vi "Query Max Current Limit.vi"(8 "error in (no error)":errorcluster, 9 "voltage level (0.0 Volts)":dbl[unit] format="%^.2e", 10 "channel name (\"CHANNEL1\")":string="CHANNEL1", 11 "IVI_DCPwr in":refnum<class "IVI_DCPwr.lvclass">) -> (0 "error out":errorcluster, 2 "max current limit":dbl[unit] format="%^.2e", 3 "IVI_DCPwr out":refnum<class "IVI_DCPwr.lvclass">)   [LabVIEW 2013, in "IVI_DCPwr.lvlib" / "IVI_DCPwr.lvclass"]
doc: "This VI returns the maximum programmable current limit that the power supply accepts for a particular voltage level on a channel for the output range to which the power supply is currently configured."
uses:
  IVI_DCPwr.lvclass
  IVI_DCPwr.lvclass/IVI_DCPwr.ctl
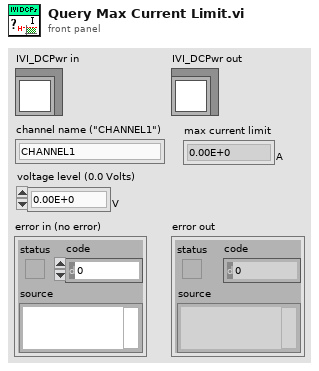
[diagram p1: front panel]
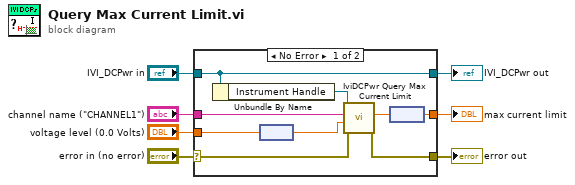
[diagram p0: block diagram]
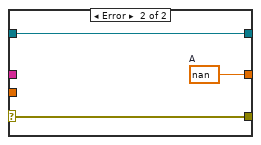
[diagram p2: hidden frame]
diagram:
  n1 = case shown="No Error" "error in (no error)" {
    selector: "error in (no error)" -> [w14 w19]
    tunnel: [w13 w19] -> w6
    tunnel: [w16 w18] -> w4
    tunnel: "IVI_DCPwr in" -> [w16 w18]
    tunnel: "channel name (\"CHANNEL1\")" -> [w12 _]
    tunnel: [w8 w17] -> w1
    tunnel: "voltage level (0.0 Volts)" -> [w10 _]
    frame No Error {
      n2 = Unbundle By Name(w16) -> ("Instrument Handle"=w15:refnum<k15>)
      n3 = node(w10) -> (w9:dbl)
      n4 = call <vilib>:"IviDCPwr Query Max Current Limit.vi"("error in (no error)"=w14, "voltage level (0.0 Volts)"=w9, "channel name (\"CHANNEL1\")"=w12, "instrument handle"=w15) -> ("error out"=w13:errorcluster, "max current limit"=w11:dbl)  [unwired: 5 in, 1 out]
      n5 = node(w11) -> (w8:dbl[unit])
    }
    frame Error {
      w17 = dbl[unit] nan  # A
    }
  }
  "error out" <- w6
  "IVI_DCPwr out" <- w4
  "max current limit" <- w1
